vi "motor_direction.vi"(9 "y":dbl, 10 "degree":dbl, 11 "x":dbl) -> (1 "direction out":dbl[](array[numeric]))   [LabVIEW 2019]
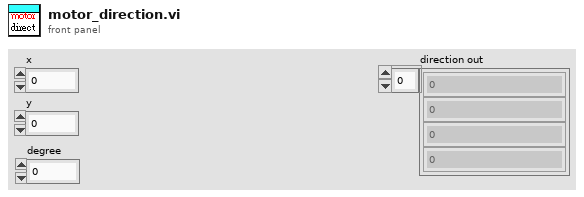
[diagram p1: front panel]
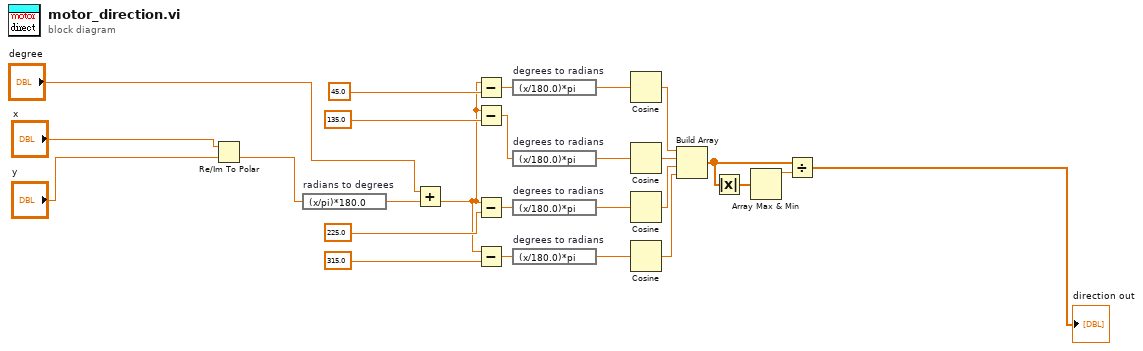
[diagram p0: block diagram]
diagram:
  n1 = Re/Im To Polar(2:"y", 3:"x") -> (0:w1:dbl)  [unwired: 1 out]
  n2 = expression code="(x/pi)*180.0" "radians to degrees"(w1) -> (w8:dbl)
  n3 = Add(x="degree", y=w8) -> (x+y=w6:dbl)
  n4 = Subtract(x=w6, y=45.0 ("x")) -> (x-y=w16:dbl)
  n5 = Subtract(x=w6, y=135.0) -> (x-y=w15:dbl)
  n6 = Subtract(x=w6, y=225.0) -> (x-y=w14:dbl)
  n7 = Subtract(x=w6, y=315.0) -> (x-y=w13:dbl)
  n8 = expression code="(x/180.0)*pi" "degrees to radians"(w16) -> (w25:dbl)
  n9 = expression code="(x/180.0)*pi" "degrees to radians"(w15) -> (w23:dbl)
  n10 = expression code="(x/180.0)*pi" "degrees to radians"(w14) -> (w17:dbl)
  n11 = expression code="(x/180.0)*pi" "degrees to radians"(w13) -> (w18:dbl)
  n12 = Cosine(x=w25) -> (cos(x)=w26:dbl)
  n13 = Cosine(x=w23) -> (cos(x)=w24:dbl)
  n14 = Cosine(x=w17) -> (cos(x)=w22:dbl)
  n15 = Cosine(x=w18) -> (cos(x)=w21:dbl)
  n16 = Build Array(w26, w24, w22, w21) -> (w19:dbl[])
  n17 = Absolute Value(x=w19) -> (abs(x)=w7:dbl[])
  n18 = Array Max & Min(array=w7) -> (max value=w20:dbl)  [unwired: 3 out]
  n19 = Divide(x=w19, y=w20) -> (x/y=→"direction out":dbl[])
